vi "Finish.vi"   [LabVIEW 2015]
doc: "This VI is called just before exiting. It is expected to close I/O refnum, save collected data, etc."
uses:
  <vilib>/Rock Robotics/WPI/Utilities/WPI_GetSetVariantRefNum.vi
  <instrlib>/navX Library v2/navX Library v2.lvlib
types:
  T1 = typedef "WPI_JoystickDevRef.ctl" = cluster{"Device":T2}
  T2 = typedef "WPI_JoystickDeviceEnum.ctl" = enum16{"USB 0", "USB 1", "USB 2", "USB 3", "USB 4", "USB 5"}
  T3 = typedef "WPI_RobotDriveDevRef.ctl" = cluster{"DevStatus":errorcluster, "Motors[]":T4[], "Square Inputs":bool, "Max Output":dbl}
  T4 = typedef "WPI_MotorControlDeviceRef.ctl" = cluster{"DeviceStatus":errorcluster, "Type":T5, "PWM":cluster{"PWM Channel":T6, "DeadBand":T7}, "CAN":cluster{"Device Number":u8, "Control Mode":T8, "Semaphore":T9, "Max Vout":dbl, "TalonSRX Control Mode":T10}, "Invert":bool}
  T5 = typedef "WPI_MotorControlType.ctl" = enum16{"PWM", "CAN", "CANTalonSRX"}
  T6 = typedef "FPGA_DIOPWMChannel.ctl" = enum8{"PWM 0", "PWM 1", "PWM 2", "PWM 3", "PWM 4", "PWM 5", "PWM 6", "PWM 7", "PWM 8", "PWM 9", "PWM MXP 0", "PWM MXP 1", "PWM MXP 2", "PWM MXP 3", "PWM MXP 4", "PWM MXP 5", "PWM MXP 6", "PWM MXP 7", "PWM MXP 8", "PWM MXP 9", "Invalid"}
  T7 = typedef "WPI_PWMDeadband.ctl" = cluster{"Name":string, "maxPositivePwm":i32, "minPositivePwm":i32, "centerPwm":i32, "maxNegativePwm":i32, "minNegativePwm":i32, "angularRange":u16}
  T8 = typedef "WPI_CANJaguar_ControlMode.ctl" = enum8{"Percent VBus", "Current", "Speed", "Position", "Voltage"}
  T9 = typedef "Semaphore RefNum" = refnum<k1>
  T10 = typedef "WPI_CANTalonSRX_APIControlMode.ctl" = enum8{"Percent VBus", "Speed", "Position", "Slave", "Unchanged / Invalid", "Voltage Compensation", "Current", "Motion Profile"}
  T11 = typedef "WPI_SolenoidDevRef.ctl" = cluster{"DevStatus":errorcluster, "Pneumatics Control Module":u8, "Forward Solenoid Channel":T12, "Reverse Solenoid Channel":T12}
  T12 = typedef "WPI_SolenoidChannel.ctl" = enum8{"Solenoid 0", "Solenoid 1", "Solenoid 2", "Solenoid 3", "Solenoid 4", "Solenoid 5", "Solenoid 6", "Solenoid 7", "Invalid"}
  T13 = typedef "navX Library v2.lvlib/Z900_navX_DeviceTypeDef.ctl" = cluster{"Interface":cluster{"Protocol":T14, "Update Rate (4Hz-60Hz)":u8, "navX Open TypeDef":variant}, "Notify Packet":refnum<notifier>, "Loop VI Refnum":refnum<vi>, "Ready to Close Occurrence Refnum":refnum<k4>}
  T14 = typedef "navX Library v2.lvlib/Z900_navX_ProtocolTypeDef.ctl" = enum16{"SERIAL", "I2C", "SPI"}
  T15 = typedef "WPI_EncoderDevRef.ctl" = cluster{"DevStatus":errorcluster, "EncoderIndex":T16, "CounterIndex":T17, "DistancePerCount":dbl, "Decoding Type":T18}
  T16 = typedef "FPGA_EncoderIdx.ctl" = enum8{"Enc 0", "Enc 1", "Enc 2", "Enc 3", "Enc 4", "Enc 5", "Enc 6", "Enc 7", "Invalid"}
  T17 = typedef "FPGA_CounterCtrSystemIndex.ctl" = enum8{"Ctr 0", "Ctr 1", "Ctr 2", "Ctr 3", "Ctr 4", "Ctr 5", "Ctr 6", "Ctr 7", "Invalid"}
  T18 = typedef "WPI_EncoderType.ctl" = enum16{"1x", "2x", "4x"}
  T19 = typedef "WPI_SwitchDevRef.ctl" = cluster{"DevStatus":errorcluster, "DIO Channel":T20, "CntIndex":T17, "Normally Closed":bool}
  T20 = typedef "FPGA_DIOChannel.ctl" = enum8{"DIO 0", "DIO 1", "DIO 2", "DIO 3", "DIO 4", "DIO 5", "DIO 6", "DIO 7", "DIO 8", "DIO 9", "DIO MXP 0", "DIO MXP 1", "DIO MXP 2", "DIO MXP 3", "DIO MXP 4", "DIO MXP 5", "DIO MXP 6", "DIO MXP 7", "DIO MXP 8", "DIO MXP 9", "DIO MXP 10", "DIO MXP 11", "DIO MXP 12", "DIO MXP 13", "DIO MXP 14", "DIO MXP 15", "Invalid"}
  T21 = typedef "WPI_DigitalInputDevRef.ctl" = cluster{"DevStatus":errorcluster, "DIO Channel":T20}
  T22 = typedef "WPI_RelayDevRef.ctl" = cluster{"DevStatus":errorcluster, "Relay Channel":T23, "Relay Direction":T24}
  T23 = typedef "FPGA_DIORelayChannel.ctl" = enum8{"Relay 0", "Relay 1", "Relay 2", "Relay 3", "Invalid"}
  T24 = typedef "WPI_RelayDirection.ctl" = enum16{"Both directions", "Forward only", "Reverse only"}
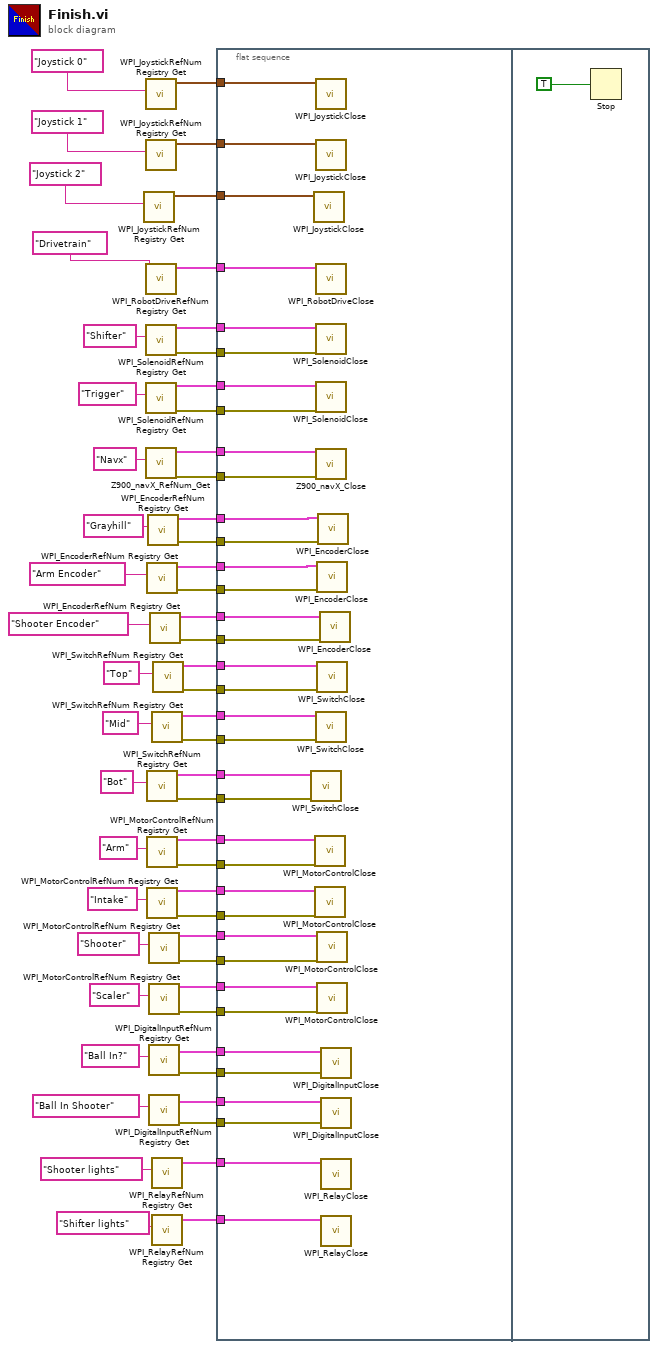
[diagram p0: block diagram]
diagram:
  n1 = call <vilib>:"WPI_JoystickRefNum Registry Get.vi"("refnum name"="Joystick 2") -> ("JoystickDevRef"=w50:T1)  [unwired: 1 in, 9 out]
  n2 = call <vilib>:"WPI_JoystickRefNum Registry Get.vi"("refnum name"="Joystick 0") -> ("JoystickDevRef"=w54:T1)  [unwired: 1 in, 9 out]
  n3 = call <vilib>:"WPI_JoystickRefNum Registry Get.vi"("refnum name"="Joystick 1") -> ("JoystickDevRef"=w53:T1)  [unwired: 1 in, 9 out]
  n4 = call <vilib>:"WPI_RobotDriveRefNum Registry Get.vi"("refnum name"="Drivetrain") -> ("RobotDriveDevRef"=w55:T3)  [unwired: 1 in, 9 out]
  n5 = call <vilib>:"WPI_SolenoidRefNum Registry Get.vi"("refnum name"="Shifter") -> ("error out"=w48:errorcluster, "SolenoidDevRef"=w49:T11)  [unwired: 9 in]
  n6 = call <vilib>:"WPI_SolenoidRefNum Registry Get.vi"("refnum name"="Trigger") -> ("error out"=w45:errorcluster, "SolenoidDevRef"=w44:T11)  [unwired: 9 in]
  n7 = call <instrlib>:"Z900_navX_RefNum_Get.vi"("refnum name"="Navx") -> ("error out"=w42:errorcluster, "navX Device"=w43:T13)  [unwired: 9 in]
  n8 = call <vilib>:"WPI_EncoderRefNum Registry Get.vi"("refnum name"="Arm Encoder") -> ("error out"=w36:errorcluster, "EncoderDevRef"=w35:T15)  [unwired: 9 in]
  n9 = call <vilib>:"WPI_SwitchRefNum Registry Get.vi"("refnum name"="Bot") -> ("error out"=w24:errorcluster, "SwitchDevRef"=w25:T19)  [unwired: 9 in]
  n10 = call <vilib>:"WPI_MotorControlRefNum Registry Get.vi"("refnum name"="Arm") -> ("error out"=w21:errorcluster, "MotorControlDevRef"=w22:T4)  [unwired: 9 in]
  n11 = call <vilib>:"WPI_MotorControlRefNum Registry Get.vi"("refnum name"="Intake") -> ("error out"=w18:errorcluster, "MotorControlDevRef"=w17:T4)  [unwired: 9 in]
  n12 = call <vilib>:"WPI_EncoderRefNum Registry Get.vi"("refnum name"="Grayhill") -> ("error out"=w39:errorcluster, "EncoderDevRef"=w40:T15)  [unwired: 9 in]
  n13 = call <vilib>:"WPI_MotorControlRefNum Registry Get.vi"("refnum name"="Shooter") -> ("error out"=w15:errorcluster, "MotorControlDevRef"=w16:T4)  [unwired: 9 in]
  n14 = call <vilib>:"WPI_MotorControlRefNum Registry Get.vi"("refnum name"="Scaler") -> ("error out"=w12:errorcluster, "MotorControlDevRef"=w11:T4)  [unwired: 9 in]
  n15 = call <vilib>:"WPI_DigitalInputRefNum Registry Get.vi"("refnum name"="Ball In?") -> ("error out"=w9:errorcluster, "DigitalInputDevRef"=w10:T21)  [unwired: 9 in]
  n16 = call <vilib>:"WPI_DigitalInputRefNum Registry Get.vi"("refnum name"="Ball In Shooter") -> ("error out"=w6:errorcluster, "DigitalInputDevRef"=w5:T21)  [unwired: 9 in]
  n17 = call <vilib>:"WPI_EncoderRefNum Registry Get.vi"("refnum name"="Shooter Encoder") -> ("error out"=w33:errorcluster, "EncoderDevRef"=w34:T15)  [unwired: 9 in]
  n18 = call <vilib>:"WPI_SwitchRefNum Registry Get.vi"("refnum name"="Mid") -> ("error out"=w27:errorcluster, "SwitchDevRef"=w26:T19)  [unwired: 9 in]
  n19 = call <vilib>:"WPI_RelayRefNum Registry Get.vi"("refnum name"="Shooter lights") -> ("RelayDevRef"=w3:T22)  [unwired: 9 in, 1 out]
  n20 = call <vilib>:"WPI_RelayRefNum Registry Get.vi"("refnum name"="Shifter lights") -> ("RelayDevRef"=w2:T22)  [unwired: 9 in, 1 out]
  n21 = call <vilib>:"WPI_SwitchRefNum Registry Get.vi"("refnum name"="Top") -> ("error out"=w30:errorcluster, "SwitchDevRef"=w31:T19)  [unwired: 9 in]
  n22 = flat-sequence {
    tunnel: w55 -> [w93]
    tunnel: w54 -> [w92]
    tunnel: w53 -> [w91]
    tunnel: w50 -> [w90]
    tunnel: w49 -> [w89]
    tunnel: w48 -> [w88]
    tunnel: w44 -> [w86]
    tunnel: w45 -> [w87]
    tunnel: w43 -> [w85]
    tunnel: w42 -> [w84]
    tunnel: w40 -> [w83]
    tunnel: w39 -> [w82]
    tunnel: w35 -> [w80]
    tunnel: w36 -> [w81]
    tunnel: w34 -> [w78]
    tunnel: w33 -> [w79]
    tunnel: w31 -> [w77]
    tunnel: w30 -> [w76]
    tunnel: w26 -> [w74]
    tunnel: w27 -> [w75]
    tunnel: w25 -> [w73]
    tunnel: w24 -> [w72]
    tunnel: w22 -> [w71]
    tunnel: w21 -> [w70]
    tunnel: w17 -> [w68]
    tunnel: w18 -> [w69]
    tunnel: w16 -> [w67]
    tunnel: w15 -> [w66]
    tunnel: w11 -> [w64]
    tunnel: w12 -> [w65]
    tunnel: w10 -> [w63]
    tunnel: w9 -> [w62]
    tunnel: w5 -> [w60]
    tunnel: w6 -> [w61]
    tunnel: w3 -> [w59]
    tunnel: w2 -> [w58]
    frame #0 {
      n23 = call <vilib>:"WPI_SwitchClose.vi"("error in (no error)"=w72, "SwitchDevRef"=w73) -> ()  [unwired: 9 in, 1 out]
      n24 = call <vilib>:"WPI_JoystickClose.vi"("JoystickDevRef"=w90) -> ()  [unwired: 11 out]
      n25 = call <vilib>:"WPI_MotorControlClose.vi"("error in (no error)"=w70, "MotorControlDevRef"=w71) -> ()  [unwired: 9 in, 1 out]
      n26 = call <vilib>:"WPI_MotorControlClose.vi"("error in (no error)"=w69, "MotorControlDevRef"=w68) -> ()  [unwired: 9 in, 1 out]
      n27 = call <vilib>:"WPI_JoystickClose.vi"("JoystickDevRef"=w92) -> ()  [unwired: 11 out]
      n28 = call <vilib>:"WPI_JoystickClose.vi"("JoystickDevRef"=w91) -> ()  [unwired: 11 out]
      n29 = call <vilib>:"WPI_RobotDriveClose.vi"("RobotDriveDevRef"=w93) -> ()  [unwired: 1 in, 10 out]
      n30 = call <vilib>:"WPI_SolenoidClose.vi"("error in (no error)"=w88, "SolenoidDevRef"=w89) -> ()  [unwired: 9 in, 1 out]
      n31 = call <vilib>:"WPI_SolenoidClose.vi"("error in (no error)"=w87, "SolenoidDevRef"=w86) -> ()  [unwired: 9 in, 1 out]
      n32 = call <instrlib>:"Z900_navX_Close.vi"("error in (no error)"=w84, "navX Device"=w85) -> ()  [unwired: 9 in, 1 out]
      n33 = call <vilib>:"WPI_SwitchClose.vi"("error in (no error)"=w75, "SwitchDevRef"=w74) -> ()  [unwired: 9 in, 1 out]
      n34 = call <vilib>:"WPI_EncoderClose.vi"("error in (no error)"=w81, "EncoderDevRef"=w80) -> ()  [unwired: 9 in, 1 out]
      n35 = call <vilib>:"WPI_SwitchClose.vi"("error in (no error)"=w76, "SwitchDevRef"=w77) -> ()  [unwired: 9 in, 1 out]
      n36 = call <vilib>:"WPI_MotorControlClose.vi"("error in (no error)"=w66, "MotorControlDevRef"=w67) -> ()  [unwired: 9 in, 1 out]
      n37 = call <vilib>:"WPI_MotorControlClose.vi"("error in (no error)"=w65, "MotorControlDevRef"=w64) -> ()  [unwired: 9 in, 1 out]
      n38 = call <vilib>:"WPI_EncoderClose.vi"("error in (no error)"=w82, "EncoderDevRef"=w83) -> ()  [unwired: 9 in, 1 out]
      n39 = call <vilib>:"WPI_EncoderClose.vi"("error in (no error)"=w79, "EncoderDevRef"=w78) -> ()  [unwired: 9 in, 1 out]
      n40 = call <vilib>:"WPI_DigitalInputClose.vi"("error in (no error)"=w62, "DigitalInputDevRef"=w63) -> ()  [unwired: 9 in, 1 out]
      n41 = call <vilib>:"WPI_DigitalInputClose.vi"("error in (no error)"=w61, "DigitalInputDevRef"=w60) -> ()  [unwired: 9 in, 1 out]
      n42 = call <vilib>:"WPI_RelayClose.vi"("RelayDevRef"=w59) -> ()  [unwired: 10 in, 1 out]
      n43 = call <vilib>:"WPI_RelayClose.vi"("RelayDevRef"=w58) -> ()  [unwired: 10 in, 1 out]
    }
    frame #1 {
      n44 = Stop(stop? (T)=TRUE ("Quit")) -> ()
    }
  }
